vi "TDMS_Open_process - Copy.vi"(9 "Input 2D":dbl[][](array[numeric]), 11 "Open":bool) -> (1 "Output 2D":dbl[][](array[numeric]), 3 "Freq_Sampling_SizeX_SizeY":dbl[](array[numeric]))   [LabVIEW 2012]
uses:
  <vilib>/Analysis/Matrix/Datatypes/RealMatrix.ctl
  <vilib>/Platform/NI_3dgraph.lvlib
  <vilib>/Analysis/Matrix/NI_Matrix.lvlib
panel:
  out "sum":u32
  out "Numeric":i32
  in  "x":i32=22650
  out "size(s) 4":i32
  out "element 2":i32
  out "size(s) 3":i32[](array[numeric])
  out "chuck":dbl
  out "element":dbl
  out "Start1":dbl
  out "LEngth":dbl
  out "Start 2":dbl
  out "channel names":string[](array[string])
  out "size(s)":i32[](array[numeric])
  in  "3D Surface":refnum<k7>(container)
  in  "Gate 1":dbl
  in  "Gate 2":dbl=25.0
  in  "Samples per Channel":i32=1000 caption="Samples"
  in  "Rate":dbl=60000.0 caption="Sample Rate (Hz)" format="%0.0f"
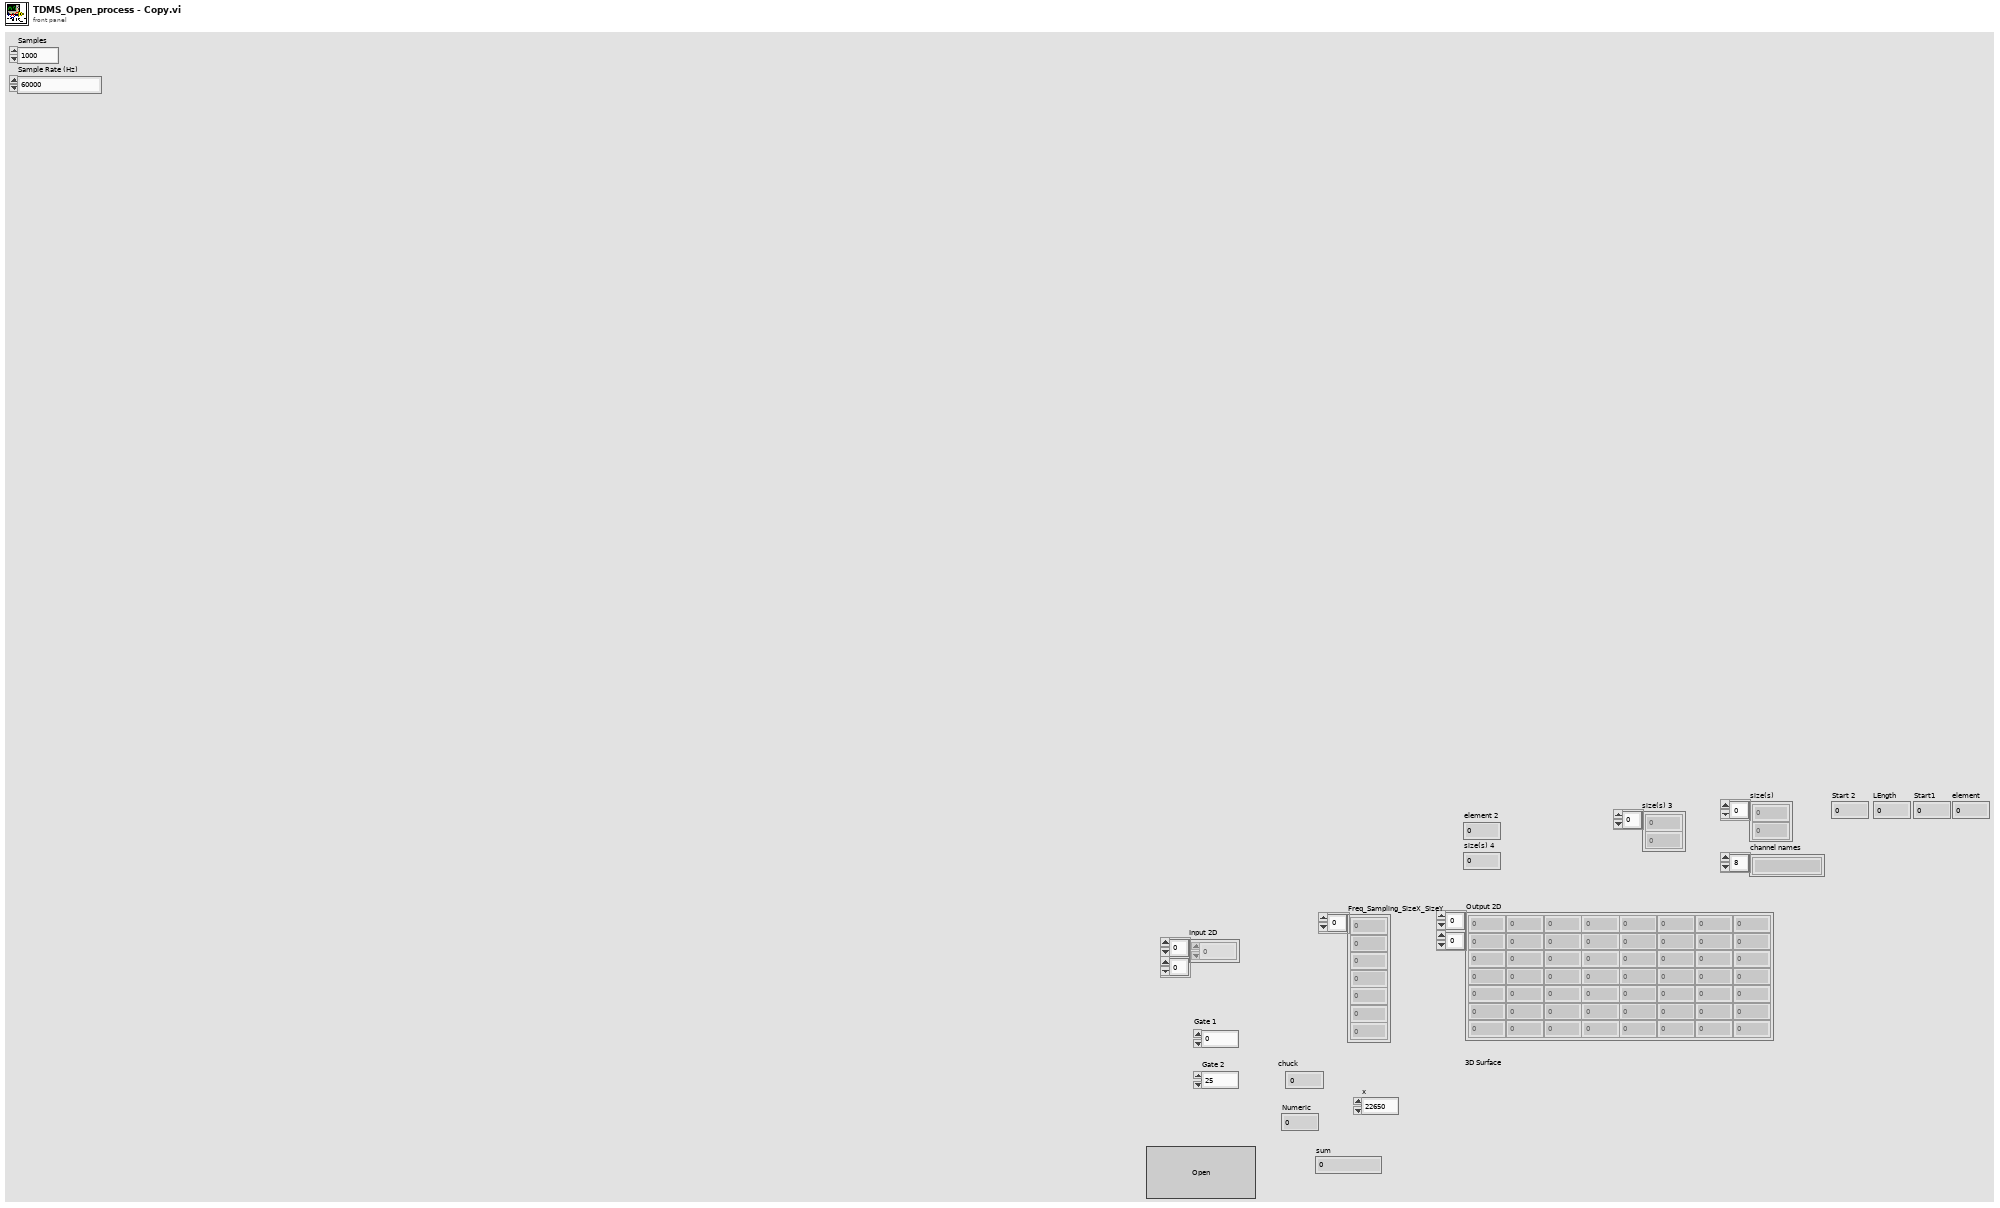
[diagram p1: front panel]
types:
  T1 = typedef "NI_Matrix.lvlib/RealMatrix.ctl" = dbl[][]
  T2 = enum16{"open", "open or create", "create or replace", "create", "open (read-only)"}
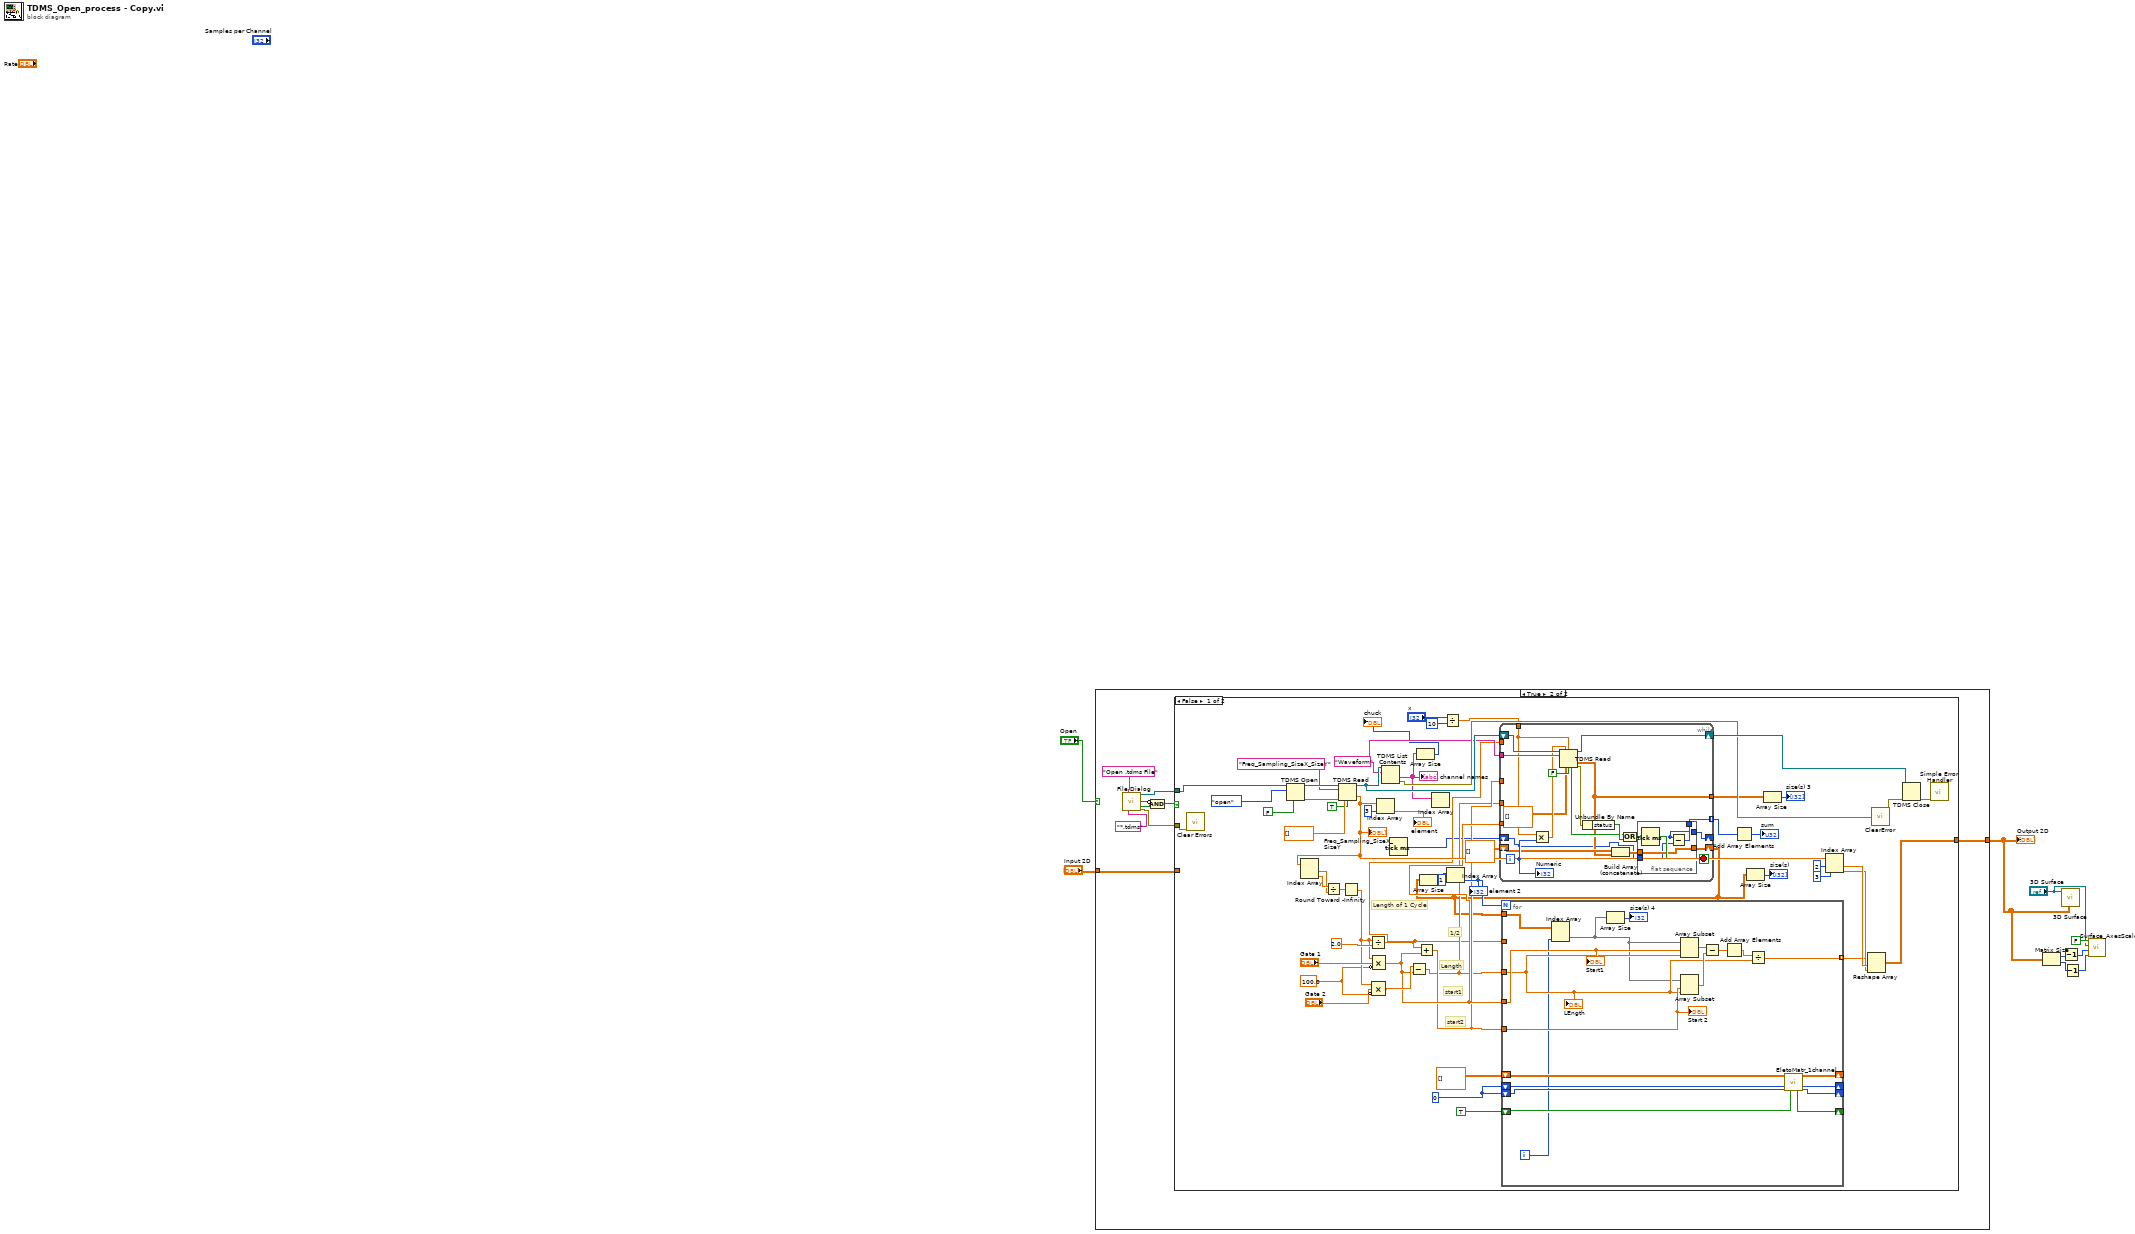
[diagram p0: block diagram]
diagram:
  n1 = case shown="True" "Open" {
    tunnel: [w10 w12] -> w2
    tunnel: "Input 2D" -> [w10 w11]
    frame False {
    }
    frame True {
      n2 = call "File Dialog"("prompt"="Open .tdms File" ("button label"), "pattern (all files)"="*.tdms") -> ("selected path"=w19:path, "exists"=w17:bool, "cancelled"=w16:bool, "error out"=w14:errorcluster)  [unwired: 10 in]
      n3 = Compound Arithmetic op=AND(invert w17, w16) -> (w15:bool)
      n4 = case shown="False" w15 {
        tunnel: w19 -> [w66 _]
        tunnel: w14 -> [w75 _]
        tunnel: [w26 w119] -> w12
        tunnel: w11 -> [_ w119]
        frame False {
          w44 = 100.0 ("蔼")
          w63 = 0 ("Out Row")
          w39 = "Waveform" ("group name in")
          # "Length of 1 Cycle"
          # "start2"
          # "1/2"
          # "start1"
          # "Length"
          n5 = call <vilib>:"Clear Errors.vi"("error in (no error)"=w75) -> ()  [unwired: 6 in, 1 out]
          n6 = TDMS Open(6:FALSE ("disable buffering (T)"), 10:T2."open" ("operation"), 11:w66) -> (0:w70:errorcluster, 3:w74:refnum<k34>)  [unwired: 3 in]
          n7 = TDMS Read(0:w74, 5:"Freq_Sampling_SizeX_SizeY" ("group name in"), 11:w70, 12:dbl[] [] ("Array"), 13:TRUE ("return channels in file order? (F)")) -> (4:w40:refnum<k34>, 10:w53:dbl[])  [unwired: 3 in, 4 out]
          "Freq_Sampling_SizeX_SizeY" <- w53
          n8 = Index Array(array=w53) -> (element #1=w59:dbl, element #2=w60:dbl)  [unwired: 2 in]
          n9 = Divide(x=w60, y=w59) -> (x/y=w61:dbl)
          n10 = Round Toward -Infinity(1:w61) -> (0:w46:dbl)
          n11 = Divide(x=w46, y=2.0) -> (x/y=w27:dbl)
          n12 = Compound Arithmetic op=MULTIPLY(w46, "Gate 2", invert w44) -> (w43:dbl)
          n13 = Compound Arithmetic op=MULTIPLY(w46, "Gate 1", invert w44) -> (w30:dbl)
          n14 = Index Array(array=w53, index=3) -> (element=→"element":dbl)
          n15 = TDMS List Contents(6:w39, 7:w40) -> (0:w41:errorcluster, 1:w35:string[])  [unwired: 1 in, 2 out]
          "channel names" <- w35
          n16 = Tick Count (ms)() -> (millisecond timer value=w22:u32)
          n17 = Subtract(x=w43, y=w30) -> (x-y=w28:dbl)
          n18 = Array Size(array=w35) -> (size(s)=→"chuck":i32)
          n19 = Add(x=w27, y=w30) -> (x+y=w29:dbl)
          n20 = Index Array(array=w35) -> ()  [unwired: 1 in, 1 out]
          n21 = Divide(x="x", y=10) -> (x/y=w36:dbl)
          n22 = while {
            tunnel: w39 -> [w93]
            shift-right: [w92] -> w58
            shift-left: w40 -> [w94]
            tunnel: w36 -> [w76]
            tunnel: [w82] -> w31
            tunnel: w30 -> [_]
            tunnel: w29 -> [_]
            tunnel: w28 -> [_]
            tunnel: w27 -> [_]
            shift-right: [w81] -> w23
            shift-left: T1 [] ("Real Matrix") -> [w83]
            shift-right: [w77] -> _
            shift-left: w22 -> [w79]
            tunnel: [w78] -> w21 mode=indexing
            i -> [w90]
            stop <- w87 stop-if-true
            n23 = Multiply(x=w76, y=w90) -> (x*y=w91:dbl)
            n24 = TDMS Read(0:w94, 1:w91, 2:w76, 5:w93, 12:dbl[][] [] ("Array"), 13:FALSE ("return channels in file order? (F)")) -> (4:w92:refnum<k34>, 10:w82:dbl[][], 14:w85:bool, 15:w88:errorcluster)  [unwired: 2 in, 2 out]
            n25 = Unbundle By Name(w88) -> ("status"=w89:bool)
            n26 = Build Array (concatenate)(w83, w82) -> (w80:T1)
            n27 = Compound Arithmetic op=OR(w85, w89) -> (w87:bool)
            n28 = flat-sequence {
              tunnel: [w98] -> w81
              tunnel: w80 -> [w98]
              tunnel: w79 -> [w97]
              tunnel: [w96] -> w78
              tunnel: [w95] -> w77
              frame #0 {
                n29 = Tick Count (ms)() -> (millisecond timer value=w95:u32)
                n30 = Subtract(x=w95, y=w97) -> (x-y=w96:u32)
              }
            }
            "Numeric" <- w90
          }
          n31 = Array Size(array=w23) -> (size(s)=w50:i32[])
          n32 = Index Array(array=w50, index=1) -> (element=w48:i32)
          "element 2" <- w48
          n33 = for {
            N: w48 -> [_]
            tunnel: w28 -> [w112]
            tunnel: w29 -> [w114]
            tunnel: w30 -> [w113]
            tunnel: w27 -> [_]
            shift-right: [w110] -> _
            shift-left: dbl[][] [] ("Out Array X") -> [w111]
            shift-right: [w109] -> _
            shift-left: w63 -> [w106]
            shift-right: [w108] -> _
            shift-left: w63 -> [w107]
            shift-right: [w104] -> _
            shift-left: TRUE ("Output Direction") -> [w105]
            tunnel: w23 -> [w103]
            tunnel: [w99] -> w25 mode=indexing
            i -> [w102]
            n34 = Index Array(array=w103, index (col)=w102) -> (element=w101:dbl[])  [unwired: 1 in]
            n35 = Array Size(array=w101) -> (size(s)=→"size(s) 4":i32)
            n36 = Array Subset(array=w101, index=w113, length=w112) -> (w117:dbl[])
            n37 = Array Subset(array=w101, index=w114, length=w112) -> (w116:dbl[])
            n38 = Subtract(x=w117, y=w116) -> (x-y=w115:dbl[])
            n39 = Add Array Elements(numeric array=w115) -> (sum=w118:dbl)
            n40 = Divide(x=w118, y=w112) -> (x/y=w99:dbl)
            n41 = call "EletoMatr_1channel.vi"("Input Array X"=w111, "In Row"=w106, "In Column"=w107, "Input Direction"=w105) -> ("Out Array X"=w110:dbl[][], "Out Row"=w109:i32, "Output Direction"=w104:bool, "Out Column"=w108:i32)  [unwired: 7 in, 1 out]
            "Start 2" <- w114
            "LEngth" <- w112
            "Start1" <- w113
          }
          n42 = Add Array Elements(numeric array=w21) -> (sum=→"sum":u32)
          n43 = Array Size(array=w23) -> (size(s)=→"size(s)":i32[])
          n44 = Array Size(array=w31) -> (size(s)=→"size(s) 3":i32[])
          n45 = Index Array(array=w53, index #1=2 ("index"), index #2=3 ("index")) -> (element #1=w52:dbl, element #2=w51:dbl)
          n46 = Reshape Array(w25, w52, w51) -> (w26:dbl[][])
          n47 = call <vilib>:"ClearError.vi"("error in (no error)"=w41) -> ("error out"=w68:errorcluster)
          n48 = TDMS Close(8:w68, 11:w58) -> (0:w67:errorcluster)  [unwired: 1 out]
          n49 = call <vilib>:"Simple Error Handler.vi"("error in (no error)"=w67) -> ()  [unwired: 1 in, 8 out]
        }
        frame True {
        }
      }
    }
  }
  "Output 2D" <- w2
  n50 = Matrix Size(0:w2) -> (1:w3:i32, 2:w4:i32)
  n51 = call <vilib>:"3D Surface.vi"("z matrix"=w2, "3D graph"="3D Surface") -> ()  [unwired: 8 in, 2 out]
  n52 = Decrement(x=w3) -> (x-1=w7:i32)
  n53 = Decrement(x=w4) -> (x-1=w6:i32)
  n54 = call "Surface_AxesScale.vi"("Y-axis Max"=w6, "X-axis max"=w7, "3D Surface"="3D Surface", "Auto Scale"=FALSE) -> ()  [unwired: 8 in]
